vi "Solar_V4.vi"() -> ()   [LabVIEW 2012]
uses:
  <vilib>/Utility/file.llb/Write To Spreadsheet File (string).vi
panel:
  out "DSSC1_WP 3":dbl
  out "DSSC1_WP 2":dbl
  out "DSSC3_WP":dbl
  out "POLYSI1_WP":dbl
  out "THINFILM1_WP":dbl
  out "DSSC1_WP":dbl
  out "THINFILM2_WP":dbl
  out "POLYSI2_WP":dbl
  out "DSSC2_WP":dbl
  out "Wind Angle":sgl(knob) scale=0.0..360.0
  out "Wind Speed Speed":i16(knob) scale=0.0..100.0
  out "?":string
  out "inside":dbl(slide) scale=-10.0..50.0
  out "outside":dbl(slide) scale=-10.0..50.0
  in  "EXIT":bool
  out "LED":bool
  in  "stop":bool
  out "Energy":dbl format="%#.3f"
  out "Power":dbl format="%#.3f"
  out "Current":dbl format="%#.3f"
  out "Voltage":dbl format="%#.3f"
  out "Energy":dbl format="%#.3f"
  out "Power":dbl format="%#.3f"
  out "Current":dbl format="%#.3f"
  out "Voltage":dbl format="%#.3f"
  out "Energy":dbl format="%#.3f"
  out "Power":dbl format="%#.3f"
  out "Current":dbl format="%#.3f"
  out "Voltage":dbl format="%#.3f"
  out "Energy":dbl format="%#.3f"
  out "Power":dbl format="%#.3f"
  out "Current":dbl format="%#.3f"
  out "Voltage":dbl format="%#.3f"
  out "Energy":dbl format="%#.3f"
  out "Power":dbl format="%#.3f"
  out "Current":dbl format="%#.3f"
  out "Voltage":dbl format="%#.3f"
  out "Energy":dbl format="%#.3f"
  out "Power":dbl format="%#.3f"
  out "Current":dbl format="%#.3f"
  out "Voltage":dbl format="%#.3f"
  out "Energy":dbl format="%#.3f"
  out "Power":dbl format="%#.3f"
  out "Current":dbl format="%#.3f"
  out "Voltage":dbl format="%#.3f"
  out "Poly Si 1":dbl=1.3668
  out "Poly Si 2":dbl=1.3668
  out "Thin film 2":dbl=1.3668
  out "thin Film 1":dbl=1.3668
  out "DSSC3":dbl=1.0
  out "DSSC 2":dbl=0.01296
  out "DSSC 1":dbl=0.375
  out "Waveform Chart":dynamicdata(graph)
  in  "Solar Related":T1(tab)
  out "Solar Tilted":dynamicdata(graph)
  out "Solar vertical":dynamicdata(graph)
  out "Solar Tracked":dynamicdata(graph)
  out "Solar Meteo":dynamicdata(graph)
  out "Solar UV":dynamicdata(graph)
  in  "TEMPERATURES":T2(tab)
  out "Temperature DSSC 1":dynamicdata(graph)
  out "Temperature DSSC 2":dynamicdata(graph)
  out "Temperature Poly Si":dynamicdata(graph)
  out "Temperature Thin Film":dynamicdata(graph)
  out "Array":dbl[][](array[numeric])
  # "DSSC 1"
  # "DSSC 2"
  # "DSSC 3"
  # "Poly Si 1"
  # "Poly Si 2"
  # "Thin Film 1"
  # "Thin Film 2"
  # "Temperatures"
  # "Weather Station"
  # "DSSC 1"
  # "DSSC 2"
  # "DSSC 3"
  # "Poly Si 1"
  # "Poly Si  2"
  # "Thin Film 1"
  # "Thin Film 2"
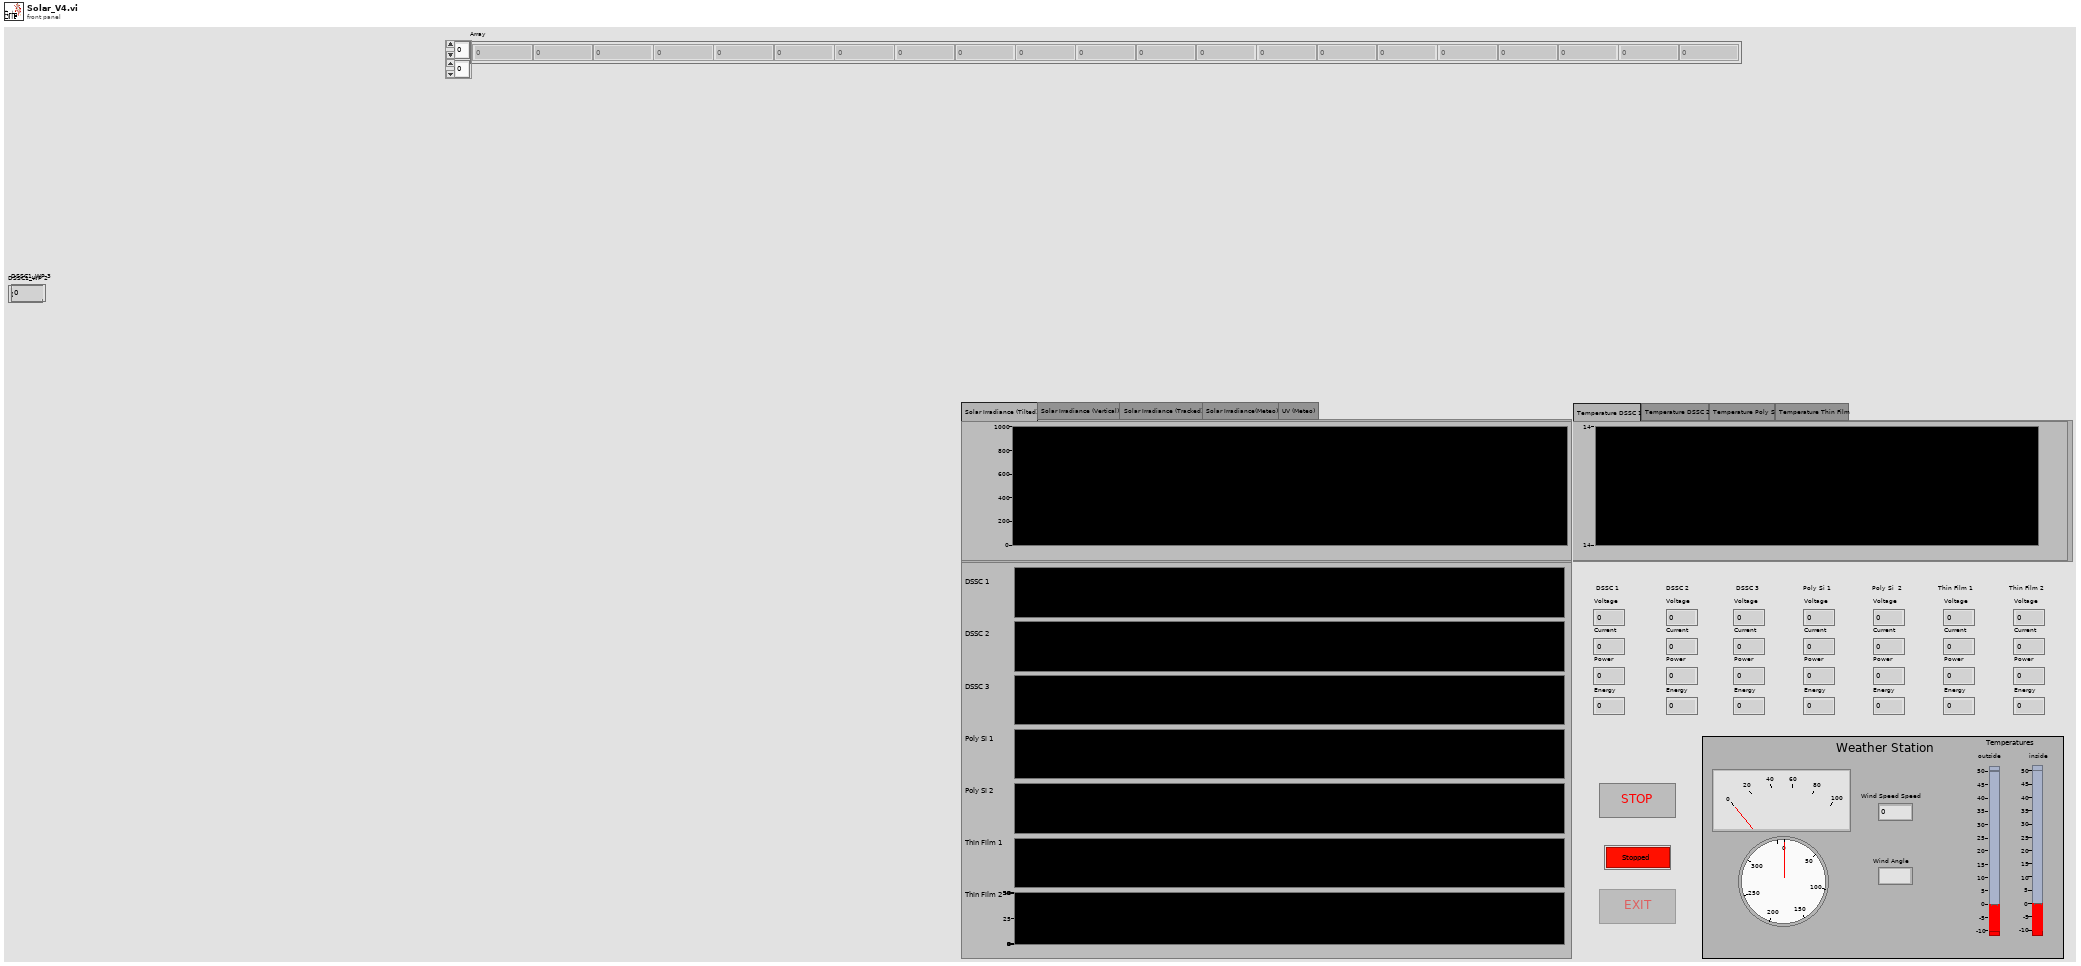
[diagram p1: front panel]
types:
  T1 = enum32{"Solar Irradiance (Tilted)", "Solar Irradiance (Vertical)", "Solar Irradiance (Tracked)", "Solar Irradiance(Meteo)", "UV (Meteo)"}
  T2 = enum32{"Temperature DSSC 1", "Temperature DSSC 2", "Temperature Poly Si", "Temperature Thin Film"}
  T3 = enum8{"Enabled", "Disabled", "Disabled and Grayed Out"}
  T4 = enum16{"open", "replace", "create", "open or create", "replace or create", "replace or create with confirmation"}
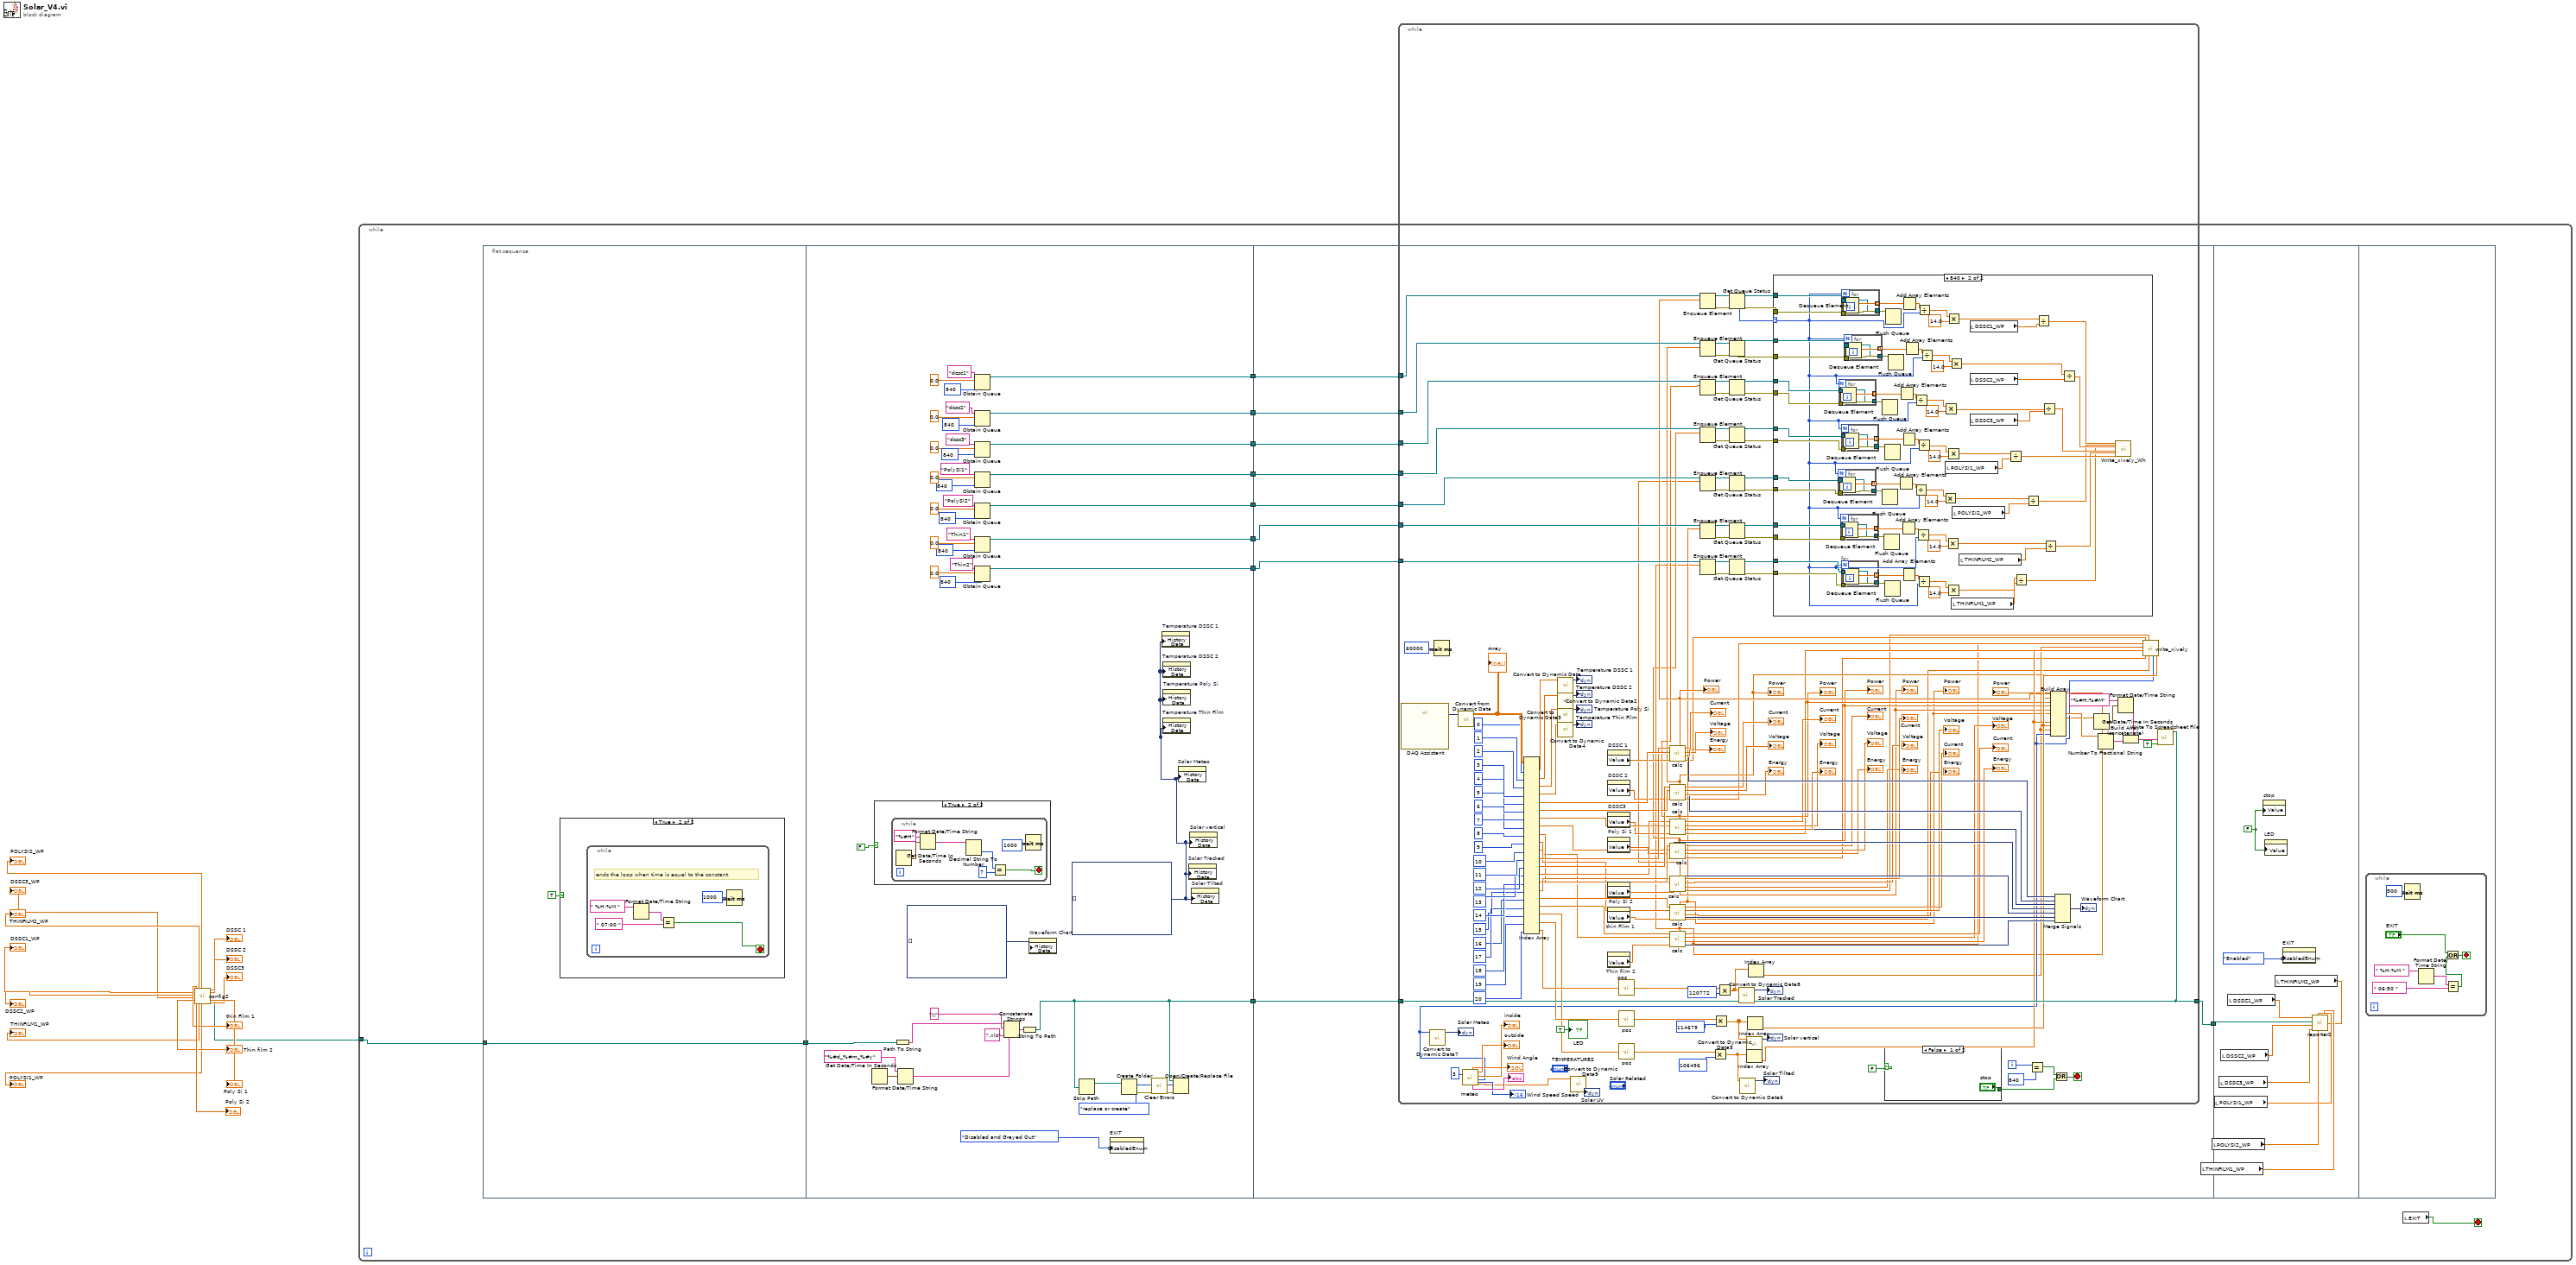
[diagram p0: block diagram]
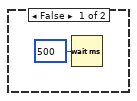
[diagram p3: hidden frame]
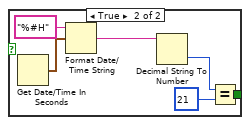
[diagram p5: hidden frame]
diagram:
  n1 = call "config2.vi"() -> ("thin Film 1"=→"thin Film 1":dbl, "DSSC1_WP"=→"DSSC1_WP":dbl, "DSSC2_WP"=→"DSSC2_WP":dbl, "DSSC3_WP"=→"DSSC3_WP":dbl, "thin Film 2"=→"Thin film 2":dbl, "Poly Si 2"=→"Poly Si 2":dbl, "THINFILM2_WP"=→"THINFILM2_WP":dbl, "THINFILM1_WP"=→"THINFILM1_WP":dbl, "POLYSI2_WP"=→"POLYSI2_WP":dbl, "POLYSI1_WP"=→"POLYSI1_WP":dbl, "Poly Si 1"=→"Poly Si 1":dbl, "DSSC 2"=→"DSSC 2":dbl, "DSSC 1"=→"DSSC 1":dbl, "path"=w8:path, "DSSC3"=→"DSSC3":dbl)  [unwired: 5 in]
  n2 = while {
    tunnel: w8 -> [w17]
    stop <- w16 stop-if-true
    n3 = flat-sequence {
      tunnel: [w29] -> w27
      tunnel: w17 -> [w29]
      tunnel: w27 -> [w38]
      tunnel: [w37] -> w26
      tunnel: [w52] -> w25
      tunnel: [w51] -> w24
      tunnel: [w50] -> w23
      tunnel: [w49] -> w22
      tunnel: [w48] -> w21
      tunnel: [w47] -> w20
      tunnel: [w46] -> w19
      tunnel: w26 -> [w96]
      tunnel: [w95] -> w18
      tunnel: w25 -> [w89]
      tunnel: w24 -> [w88]
      tunnel: w23 -> [w94]
      tunnel: w22 -> [w93]
      tunnel: w21 -> [w92]
      tunnel: w20 -> [w91]
      tunnel: w19 -> [w90]
      tunnel: w18 -> [w400]
      frame #0 {
        n4 = case shown="True" TRUE {
          frame False {
          }
          frame True {
            n5 = while {
              stop <- w30 stop-if-true
              # "ends the loop when time is equal to the constant"
              n6 = Format Date/Time String(time format string (%c)=" %H:%M ") -> (date/time string=w31:string)  [unwired: 2 in]
              n7 = Equal?(x=w31, y=" 07:00 " ("time format string (%c)")) -> (x = y?=w30:bool)
              n8 = Wait (ms)(milliseconds to wait=u32 1000) -> ()  [unwired: 1 out]
            }
          }
        }
      }
      frame #1 {
        w35 = dynamicdata[] [] ("History Data")
        n9 = Get Date/Time In Seconds() -> (seconds since 1Jan1904=w39:timestamp)
        n10 = case shown="True" FALSE {
          frame False {
            n11 = Wait (ms)(milliseconds to wait=u32 500) -> ()  [unwired: 1 out]
          }
          frame True {
            n12 = while {
              stop <- w81 stop-if-true
              n13 = Get Date/Time In Seconds() -> (seconds since 1Jan1904=w87:timestamp)
              n14 = Format Date/Time String(time format string (%c)="%#H", seconds (now)=w87) -> (date/time string=w84:string)  [unwired: 1 in]
              n15 = Decimal String To Number(string=w84) -> (number=w83:i32)  [unwired: 2 in, 1 out]
              n16 = Equal?(x=w83, y=7) -> (x = y?=w81:bool)
              n17 = Wait (ms)(milliseconds to wait=u32 1000) -> ()  [unwired: 1 out]
            }
          }
        }
        n18 = Path To String(path=w38) -> (string=w43:string)
        n19 = Format Date/Time String(time format string (%c)="%#d_%#m_%#y", seconds (now)=w39) -> (date/time string=w41:string)  [unwired: 1 in]
        n20 = Obtain Queue(max queue size (-1, unlimited)=840, name (unnamed)="dcsc1", element data type=0.0) -> (queue out=w52:refnum<queue>)  [unwired: 2 in, 2 out]
        n21 = Obtain Queue(max queue size (-1, unlimited)=840, name (unnamed)="dcsc2", element data type=0.0) -> (queue out=w51:refnum<queue>)  [unwired: 2 in, 2 out]
        n22 = Obtain Queue(max queue size (-1, unlimited)=840, name (unnamed)="dcsc3", element data type=0.0) -> (queue out=w50:refnum<queue>)  [unwired: 2 in, 2 out]
        n23 = Obtain Queue(max queue size (-1, unlimited)=840, name (unnamed)="PolySI1", element data type=0.0) -> (queue out=w49:refnum<queue>)  [unwired: 2 in, 2 out]
        n24 = Obtain Queue(max queue size (-1, unlimited)=840, name (unnamed)="PolySI2", element data type=0.0) -> (queue out=w48:refnum<queue>)  [unwired: 2 in, 2 out]
        n25 = Obtain Queue(max queue size (-1, unlimited)=840, name (unnamed)="Thin1", element data type=0.0) -> (queue out=w47:refnum<queue>)  [unwired: 2 in, 2 out]
        n26 = Obtain Queue(max queue size (-1, unlimited)=840, name (unnamed)="Thin2", element data type=0.0) -> (queue out=w46:refnum<queue>)  [unwired: 2 in, 2 out]
        n27 = Concatenate Strings(w43, "\\" ("string"), w41, ".xls" ("string")) -> (w45:string)
        n28 = String To Path(string=w45) -> (path=w37:path)
        n29 = property on="Waveform Chart" class="WFChart (strict)"("History Data"=dynamicdata[] []) -> ()  [unwired: 2 in, 2 out]
        n30 = Strip Path(path=w37) -> (stripped path=w78:path)  [unwired: 1 out]
        n31 = property on="EXIT" class="Bool (strict)"("DisabledEnum"=T3."Disabled and Grayed Out" ("Disabled")) -> ()  [unwired: 2 in, 2 out]
        n32 = Create Folder(path (use dialog)=w78) -> (error out=w77:errorcluster)  [unwired: 2 in, 2 out]
        n33 = call <vilib>:"Clear Errors.vi"("error in (no error)"=w77) -> ("error out"=w76:errorcluster)  [unwired: 6 in]
        n34 = property on="Temperature DSSC 1" class="WFChart (strict)"("History Data"=w35) -> ()  [unwired: 2 in, 2 out]
        n35 = property on="Temperature DSSC 2" class="WFChart (strict)"("History Data"=w35) -> ()  [unwired: 2 in, 2 out]
        n36 = property on="Temperature Thin Film" class="WFChart (strict)"("History Data"=w35) -> ()  [unwired: 2 in, 2 out]
        n37 = property on="Temperature Poly Si" class="WFChart (strict)"("History Data"=w35) -> ()  [unwired: 2 in, 2 out]
        n38 = Open/Create/Replace File(file path (use dialog)=w37, error in=w76, operation (0:open)=T4."replace or create") -> ()  [unwired: 3 in, 3 out]
        n39 = property on="Solar Meteo" class="WFChart (strict)"("History Data"=w35) -> ()  [unwired: 2 in, 2 out]
        n40 = property on="Solar Tracked" class="WFChart (strict)"("History Data"=w35) -> ()  [unwired: 2 in, 2 out]
        n41 = property on="Solar vertical" class="WFChart (strict)"("History Data"=w35) -> ()  [unwired: 2 in, 2 out]
        n42 = property on="Solar Tilted" class="WFChart (strict)"("History Data"=w35) -> ()  [unwired: 2 in, 2 out]
      }
      frame #2 {
        n43 = while {
          tunnel: w96 -> [w245]
          tunnel: [w245] -> w95
          tunnel: w94 -> [w116]
          tunnel: w93 -> [w115]
          tunnel: w92 -> [w114]
          tunnel: w91 -> [w113]
          tunnel: w90 -> [w112]
          tunnel: w89 -> [w118]
          tunnel: w88 -> [w117]
          i -> [w152]
          stop <- w148 stop-if-true
          n44 = call "DAQ Assistant"() -> ("data"=w246:dynamicdata)  [unwired: 17 in, 2 out]
          n45 = Wait (ms)(milliseconds to wait=u32 60000) -> ()  [unwired: 1 out]
          n46 = call "Convert from Dynamic Data"("Dynamic Data Type"=w246) -> ("Array"=w270:dbl[][])  [unwired: 3 in]
          "Array" <- w270
          n47 = call "meteo.vi"("ComPort 2"=i16 3) -> ("Wind Speed 2"=→"Wind Speed Speed":i16, "Wind Angle 2"=→"Wind Angle":sgl, "Direction 2"=→"?":string, "Outside Temperature"=→"outside":sgl, "Inside Temp"=→"inside":sgl, "Solar"=w156:i16, "UV"=w153:sgl)
          n48 = call "Convert to Dynamic Data7"("Double"=w156) -> ("Dynamic Data Type"=→"Solar Meteo":dynamicdata)  [unwired: 3 in]
          n49 = Index Array(array=w270, index (col) #1=0 ("index (row)"), index (col) #2=1 ("index (col)"), index (col) #3=2 ("index (col)"), index (col) #4=3 ("index (col)"), index (col) #5=4 ("index (col)"), index (col) #6=5 ("index (col)"), index (col) #7=6 ("index (col)"), index (col) #8=7 ("index (col)"), index (col) #9=8 ("index (col)"), index (col) #10=9 ("index (col)"), index (col) #11=10 ("index (col)"), index (col) #12=11 ("index (col)"), index (col) #13=12 ("index (col)"), index (col) #14=13 ("index (col)"), index (col) #15=14 ("index (col)"), index (col) #16=15 ("index (col)"), index (col) #17=16 ("index (col)"), index (col) #18=17 ("index (col)"), index (col) #19=18 ("index (col)"), index (col) #20=19 ("index (col)"), index (col) #21=20 ("index (col)")) -> (element #1=w187:dbl[], element #2=w186:dbl[], element #3=w185:dbl[], element #4=w184:dbl[], element #5=w237:dbl[], element #6=w227:dbl[], element #7=w224:dbl[], element #8=w220:dbl[], element #9=w202:dbl[], element #10=w201:dbl[], element #11=w200:dbl[], element #12=w236:dbl[], element #13=w226:dbl[], element #14=w225:dbl[], element #15=w206:dbl[], element #16=w205:dbl[], element #17=w204:dbl[], element #18=w203:dbl[], element #19=w171:dbl[], element #20=w172:dbl[], element #21=w207:dbl[])  [unwired: 21 in]
          n50 = call "Convert to Dynamic Data"("Array"=w187) -> ("Dynamic Data Type"=→"Temperature DSSC 1":dynamicdata)  [unwired: 3 in]
          n51 = call "Convert to Dynamic Data2"("Array"=w186) -> ("Dynamic Data Type"=→"Temperature DSSC 2":dynamicdata)  [unwired: 3 in]
          n52 = call "Convert to Dynamic Data3"("Array"=w185) -> ("Dynamic Data Type"=→"Temperature Poly Si":dynamicdata)  [unwired: 3 in]
          n53 = call "Convert to Dynamic Data4"("Array"=w184) -> ("Dynamic Data Type"=→"Temperature Thin Film":dynamicdata)  [unwired: 3 in]
          n54 = call "Convert to Dynamic Data9"("Double"=w153) -> ("Dynamic Data Type"=→"Solar UV":dynamicdata)  [unwired: 3 in]
          n55 = property on="DSSC 1" class="DigNum (strict)"() -> ("Value"=w183:dbl)  [unwired: 2 in, 2 out]
          n56 = property on="DSSC 2" class="DigNum (strict)"() -> ("Value"=w182:dbl)  [unwired: 2 in, 2 out]
          n57 = property on="DSSC3" class="DigNum (strict)"() -> ("Value"=w181:dbl)  [unwired: 2 in, 2 out]
          n58 = property on="Poly Si 1" class="DigNum (strict)"() -> ("Value"=w178:dbl)  [unwired: 2 in, 2 out]
          n59 = property on="Poly Si 2" class="DigNum (strict)"() -> ("Value"=w177:dbl)  [unwired: 2 in, 2 out]
          n60 = property on="thin Film 1" class="DigNum (strict)"() -> ("Value"=w180:dbl)  [unwired: 2 in, 2 out]
          n61 = property on="Thin film 2" class="DigNum (strict)"() -> ("Value"=w179:dbl)  [unwired: 2 in, 2 out]
          n62 = call "pos.vi"("Input"=w207) -> ("Output"=w244:dbl[])
          n63 = call "pos.vi"("Input"=w172) -> ("Output"=w175:dbl[])
          n64 = call "pos.vi"("Input"=w171) -> ("Output"=w173:dbl[])
          n65 = call "calc.vi"("Input Current"=w236, "Input voltage"=w237, "Area factor"=w183) -> ("Waveform Chart"=w233:dynamicdata, "Power"=w109:dbl, "Current"=→"Current":dbl, "Voltage"=→"Voltage":dbl, "Energy"=→"Energy":dbl, "Power(m2)"=w108:dbl)
          "Power" <- w109
          n66 = call "calc.vi"("Input Current"=w226, "Input voltage"=w227, "Area factor"=w182) -> ("Waveform Chart"=w228:dynamicdata, "Power"=w107:dbl, "Current"=→"Current":dbl, "Voltage"=→"Voltage":dbl, "Energy"=→"Energy":dbl, "Power(m2)"=w106:dbl)
          "Power" <- w107
          n67 = call "calc.vi"("Input Current"=w225, "Input voltage"=w224, "Area factor"=w181) -> ("Waveform Chart"=w221:dynamicdata, "Power"=w105:dbl, "Current"=→"Current":dbl, "Voltage"=→"Voltage":dbl, "Energy"=→"Energy":dbl, "Power(m2)"=w104:dbl)
          "Power" <- w105
          n68 = call "calc.vi"("Input Current"=w206, "Input voltage"=w220, "Area factor"=w178) -> ("Waveform Chart"=w219:dynamicdata, "Power"=w103:dbl, "Current"=→"Current":dbl, "Voltage"=→"Voltage":dbl, "Energy"=→"Energy":dbl, "Power(m2)"=w100:dbl)
          "Power" <- w103
          n69 = call "calc.vi"("Input Current"=w205, "Input voltage"=w202, "Area factor"=w177) -> ("Waveform Chart"=w199:dynamicdata, "Power"=w102:dbl, "Current"=→"Current":dbl, "Voltage"=→"Voltage":dbl, "Energy"=→"Energy":dbl, "Power(m2)"=w101:dbl)
          "Power" <- w102
          n70 = call "calc.vi"("Input Current"=w204, "Input voltage"=w201, "Area factor"=w180) -> ("Waveform Chart"=w198:dynamicdata, "Power"=w99:dbl, "Current"=→"Current":dbl, "Voltage"=→"Voltage":dbl, "Energy"=→"Energy":dbl, "Power(m2)"=w98:dbl)
          "Power" <- w99
          n71 = call "calc.vi"("Input Current"=w203, "Input voltage"=w200, "Area factor"=w179) -> ("Waveform Chart"=w197:dynamicdata, "Power"=w97:dbl, "Current"=→"Current":dbl, "Voltage"=→"Voltage":dbl, "Energy"=→"Energy":dbl)  [unwired: 1 out]
          "Power" <- w97
          n72 = Enqueue Element(queue=w118, element=w109) -> (queue out=w120:refnum<queue>, error out=w122:errorcluster)  [unwired: 2 in, 1 out]
          n73 = Enqueue Element(queue=w117, element=w107) -> (queue out=w124:refnum<queue>, error out=w125:errorcluster)  [unwired: 2 in, 1 out]
          n74 = Enqueue Element(queue=w116, element=w105) -> (queue out=w128:refnum<queue>, error out=w129:errorcluster)  [unwired: 2 in, 1 out]
          n75 = Enqueue Element(queue=w115, element=w103) -> (queue out=w130:refnum<queue>, error out=w131:errorcluster)  [unwired: 2 in, 1 out]
          n76 = Enqueue Element(queue=w114, element=w102) -> (queue out=w132:refnum<queue>, error out=w133:errorcluster)  [unwired: 2 in, 1 out]
          n77 = Enqueue Element(queue=w113, element=w99) -> (queue out=w134:refnum<queue>, error out=w135:errorcluster)  [unwired: 2 in, 1 out]
          n78 = Enqueue Element(queue=w112, element=w97) -> (queue out=w136:refnum<queue>, error out=w137:errorcluster)  [unwired: 2 in, 1 out]
          n79 = Multiply(x=w173, y=106496) -> (x*y=w166:dbl[])
          n80 = Multiply(x=w175, y=114679) -> (x*y=w167:dbl[])
          n81 = Multiply(x=w244, y=120772) -> (x*y=w168:dbl[])
          n82 = Get Queue Status(queue=w120, error in (no error)=w122) -> (queue out=w121:refnum<queue>, error out=w123:errorcluster, # elements in queue=w119:i32)  [unwired: 1 in, 5 out]
          n83 = Get Queue Status(queue=w124, error in (no error)=w125) -> (queue out=w126:refnum<queue>, error out=w127:errorcluster)  [unwired: 1 in, 6 out]
          n84 = Get Queue Status(queue=w128, error in (no error)=w129) -> (queue out=w138:refnum<queue>, error out=w139:errorcluster)  [unwired: 1 in, 6 out]
          n85 = Get Queue Status(queue=w130, error in (no error)=w131) -> (queue out=w140:refnum<queue>, error out=w141:errorcluster)  [unwired: 1 in, 6 out]
          n86 = Get Queue Status(queue=w132, error in (no error)=w133) -> (queue out=w142:refnum<queue>, error out=w143:errorcluster)  [unwired: 1 in, 6 out]
          n87 = Get Queue Status(queue=w134, error in (no error)=w135) -> (queue out=w144:refnum<queue>, error out=w145:errorcluster)  [unwired: 1 in, 6 out]
          n88 = Get Queue Status(queue=w136, error in (no error)=w137) -> (queue out=w146:refnum<queue>, error out=w147:errorcluster)  [unwired: 1 in, 6 out]
          n89 = call "Convert to Dynamic Data8"("Array"=w168) -> ("Dynamic Data Type"=→"Solar Tracked":dynamicdata)  [unwired: 3 in]
          n90 = call "Convert to Dynamic Data6"("Array"=w166) -> ("Dynamic Data Type"=→"Solar Tilted":dynamicdata)  [unwired: 3 in]
          n91 = call "Convert to Dynamic Data5"("Array"=w167) -> ("Dynamic Data Type"=→"Solar vertical":dynamicdata)  [unwired: 3 in]
          n92 = Index Array(array=w166) -> (element=w157:dbl)  [unwired: 1 in]
          n93 = Index Array(array=w167) -> (element=w158:dbl)  [unwired: 1 in]
          n94 = Index Array(array=w168) -> (element=w110:dbl)  [unwired: 1 in]
          n95 = case shown="840" w119 {
            selector: w119 -> [_ w292]
            tunnel: w121 -> [_ w348]
            tunnel: w123 -> [_ w344]
            tunnel: w126 -> [_ w334]
            tunnel: w127 -> [_ w333]
            tunnel: w138 -> [_ w302]
            tunnel: w139 -> [_ w301]
            tunnel: w140 -> [_ w300]
            tunnel: w141 -> [_ w299]
            tunnel: w142 -> [_ w298]
            tunnel: w143 -> [_ w297]
            tunnel: w144 -> [_ w296]
            tunnel: w145 -> [_ w295]
            tunnel: w146 -> [_ w294]
            tunnel: w147 -> [_ w293]
            frame 0, Default {
            }
            frame 840 {
              n96 = for {
                N: w292 -> [_]
                tunnel: w298 -> [w363]
                tunnel: [w362] -> w320 mode=indexing
                tunnel: [w361] -> w319
                tunnel: [w360] -> w318
                tunnel: w297 -> [w359]
                n97 = Dequeue Element(queue=w363, error in (no error)=w359) -> (queue out=w360:refnum<queue>, element=w362:dbl, error out=w361:errorcluster)  [unwired: 1 in, 1 out]
              }
              n98 = for {
                N: w292 -> [_]
                tunnel: w302 -> [w373]
                tunnel: [w372] -> w332 mode=indexing
                tunnel: [w371] -> w331
                tunnel: [w370] -> w330
                tunnel: w301 -> [w369]
                n99 = Dequeue Element(queue=w373, error in (no error)=w369) -> (queue out=w370:refnum<queue>, element=w372:dbl, error out=w371:errorcluster)  [unwired: 1 in, 1 out]
              }
              n100 = for {
                N: w292 -> [_]
                tunnel: w296 -> [w358]
                tunnel: [w357] -> w314 mode=indexing
                tunnel: [w356] -> w313
                tunnel: [w355] -> w312
                tunnel: w295 -> [w354]
                n101 = Dequeue Element(queue=w358, error in (no error)=w354) -> (queue out=w355:refnum<queue>, element=w357:dbl, error out=w356:errorcluster)  [unwired: 1 in, 1 out]
              }
              n102 = for {
                N: w292 -> [_]
                tunnel: w300 -> [w368]
                tunnel: [w367] -> w326 mode=indexing
                tunnel: [w366] -> w325
                tunnel: [w365] -> w324
                tunnel: w299 -> [w364]
                n103 = Dequeue Element(queue=w368, error in (no error)=w364) -> (queue out=w365:refnum<queue>, element=w367:dbl, error out=w366:errorcluster)  [unwired: 1 in, 1 out]
              }
              n104 = for {
                N: w292 -> [_]
                tunnel: w294 -> [w353]
                tunnel: [w352] -> w308 mode=indexing
                tunnel: [w351] -> w307
                tunnel: [w350] -> w306
                tunnel: w293 -> [w349]
                n105 = Dequeue Element(queue=w353, error in (no error)=w349) -> (queue out=w350:refnum<queue>, element=w352:dbl, error out=w351:errorcluster)  [unwired: 1 in, 1 out]
              }
              n106 = for {
                N: w292 -> [_]
                tunnel: w348 -> [w383]
                tunnel: [w382] -> w347 mode=indexing
                tunnel: [w381] -> w346
                tunnel: [w380] -> w345
                tunnel: w344 -> [w379]
                n107 = Dequeue Element(queue=w383, error in (no error)=w379) -> (queue out=w380:refnum<queue>, element=w382:dbl, error out=w381:errorcluster)  [unwired: 1 in, 1 out]
              }
              n108 = for {
                N: w292 -> [_]
                tunnel: w334 -> [w378]
                tunnel: [w377] -> w340 mode=indexing
                tunnel: [w376] -> w339
                tunnel: [w375] -> w338
                tunnel: w333 -> [w374]
                n109 = Dequeue Element(queue=w378, error in (no error)=w374) -> (queue out=w375:refnum<queue>, element=w377:dbl, error out=w376:errorcluster)  [unwired: 1 in, 1 out]
              }
              n110 = Flush Queue(queue=w318, error in (no error)=w319) -> ()  [unwired: 3 out]
              n111 = Flush Queue(queue=w330, error in (no error)=w331) -> ()  [unwired: 3 out]
              n112 = Flush Queue(queue=w312, error in (no error)=w313) -> ()  [unwired: 3 out]
              n113 = Flush Queue(queue=w324, error in (no error)=w325) -> ()  [unwired: 3 out]
              n114 = Flush Queue(queue=w306, error in (no error)=w307) -> ()  [unwired: 3 out]
              n115 = Flush Queue(queue=w345, error in (no error)=w346) -> ()  [unwired: 3 out]
              n116 = Flush Queue(queue=w338, error in (no error)=w339) -> ()  [unwired: 3 out]
              n117 = Add Array Elements(numeric array=w320) -> (sum=w317:dbl)
              n118 = Add Array Elements(numeric array=w332) -> (sum=w329:dbl)
              n119 = Add Array Elements(numeric array=w314) -> (sum=w311:dbl)
              n120 = Add Array Elements(numeric array=w326) -> (sum=w323:dbl)
              n121 = Add Array Elements(numeric array=w308) -> (sum=w305:dbl)
              n122 = Add Array Elements(numeric array=w347) -> (sum=w343:dbl)
              n123 = Add Array Elements(numeric array=w340) -> (sum=w337:dbl)
              n124 = Divide(x=w317, y=w292) -> (x/y=w316:dbl)
              n125 = Divide(x=w329, y=w292) -> (x/y=w328:dbl)
              n126 = Divide(x=w311, y=w292) -> (x/y=w310:dbl)
              n127 = Divide(x=w323, y=w292) -> (x/y=w322:dbl)
              n128 = Divide(x=w305, y=w292) -> (x/y=w304:dbl)
              n129 = Divide(x=w343, y=w292) -> (x/y=w342:dbl)
              n130 = Divide(x=w337, y=w292) -> (x/y=w336:dbl)
              n131 = Multiply(x=w316, y=14.0) -> (x*y=w279:dbl)
              n132 = Multiply(x=w328, y=14.0) -> (x*y=w285:dbl)
              n133 = local read "POLYSI1_WP"() -> (w280:dbl)
              n134 = Multiply(x=w310, y=14.0) -> (x*y=w276:dbl)
              n135 = Multiply(x=w322, y=14.0) -> (x*y=w282:dbl)
              n136 = Multiply(x=w304, y=14.0) -> (x*y=w272:dbl)
              n137 = Multiply(x=w342, y=14.0) -> (x*y=w291:dbl)
              n138 = Multiply(x=w336, y=14.0) -> (x*y=w288:dbl)
              n139 = local read "THINFILM1_WP"() -> (w273:dbl)
              n140 = local read "POLYSI2_WP"() -> (w277:dbl)
              n141 = local read "THINFILM2_WP"() -> (w274:dbl)
              n142 = local read "DSSC1_WP"() -> (w289:dbl)
              n143 = local read "DSSC2_WP"() -> (w286:dbl)
              n144 = local read "DSSC3_WP"() -> (w284:dbl)
              n145 = Divide(x=w282, y=w280) -> (x/y=w281:dbl)
              n146 = Divide(x=w272, y=w273) -> (x/y=w271:dbl)
              n147 = Divide(x=w279, y=w277) -> (x/y=w278:dbl)
              n148 = Divide(x=w291, y=w289) -> (x/y=w290:dbl)
              n149 = Divide(x=w285, y=w284) -> (x/y=w283:dbl)
              n150 = Divide(x=w276, y=w274) -> (x/y=w275:dbl)
              n151 = Divide(x=w288, y=w286) -> (x/y=w287:dbl)
              n152 = call "Write_xively_Wh.vi"("thinfilm2"=w271, "Thinfilm1"=w275, "Poly Si 2"=w278, "Poly Si 1"=w281, "DSSC3"=w283, "DSSC2"=w287, "DSSC1"=w290) -> ()  [unwired: 5 in]
            }
          }
          n153 = case shown="False" FALSE {
            tunnel: ["stop" w385] -> w149
            frame False {
            }
            frame True {
              n154 = Get Date/Time In Seconds() -> (seconds since 1Jan1904=w390:timestamp)
              n155 = Format Date/Time String(time format string (%c)="%#H", seconds (now)=w390) -> (date/time string=w388:string)  [unwired: 1 in]
              n156 = Decimal String To Number(string=w388) -> (number=w387:i32)  [unwired: 2 in, 1 out]
              n157 = Equal?(x=w387, y=21) -> (x = y?=w385:bool)
            }
          }
          n158 = Equal?(x=w152, y=840) -> (x = y?=w150:bool)
          n159 = Build Array(w109, w107, w105, w103, w102, w99, w97, w157, w158, w110, w156) -> (w249:dbl[])
          n160 = Or(x=w150, y=w149) -> (x .or. y?=w148:bool)
          n161 = Merge Signals(w233, w228, w221, w219, w199, w198, w197) -> (→"Waveform Chart":dynamicdata)
          n162 = Get Date/Time In Seconds() -> (seconds since 1Jan1904=w253:timestamp)
          n163 = Number To Fractional String(number=w249) -> (F-format string=w250:string[])  [unwired: 3 in]
          n164 = Format Date/Time String(time format string (%c)="%#H:%#M", seconds (now)=w253) -> (date/time string=w251:string)  [unwired: 1 in]
          n165 = Build Array (concatenate)(w251, w250) -> (w248:string[])
          n166 = call "write_xively.vi"("Solar__Tilted_"=w157, "Solar__Tracked_"=w110, "Solar__Vertical_"=w158, "Solar__meteo_"=w156, "Thin_Film_2"=w97, "Thin_Film_1"=w98, "Poly Si 2"=w101, "Poly Si 1"=w100, "DSSC3"=w104, "DSSC2"=w106, "DSSC1"=w108) -> ()  [unwired: 1 in]
          n167 = call-poly <vilib>:"Write To Spreadsheet File.vi"("append to file? (new file:F)"=TRUE, "1D data"=w248, "file path (dialog if empty)"=w245) -> ()  [unwired: 5 in, 1 out]
          "LED" <- TRUE
        }
      }
      frame #3 {
        w398 = FALSE ("stop")
        n168 = local read "THINFILM1_WP"() -> (w392:dbl)
        n169 = local read "POLYSI2_WP"() -> (w394:dbl)
        n170 = local read "POLYSI1_WP"() -> (w395:dbl)
        n171 = local read "DSSC3_WP"() -> (w393:dbl)
        n172 = local read "DSSC2_WP"() -> (w396:dbl)
        n173 = local read "DSSC1_WP"() -> (w397:dbl)
        n174 = property on="stop" class="Bool (strict)"("Value"=w398) -> ()  [unwired: 2 in, 2 out]
        n175 = property on="LED" class="Bool (strict)"("Value"=w398) -> ()  [unwired: 2 in, 2 out]
        n176 = local read "THINFILM2_WP"() -> (w391:dbl)
        n177 = property on="EXIT" class="Bool (strict)"("DisabledEnum"=T3."Enabled" ("Disabled")) -> ()  [unwired: 2 in, 2 out]
        n178 = call "reporter2.vi"("DSSC1_Wp"=w397, "PolySI1_wp"=w395, "file path (dialog if empty)"=w400, "DSSC2_WP"=w396, "Polysi2_wp"=w394, "DSSC3_Wp"=w393, "Thin1Wp"=w392, "Thin2Wp"=w391) -> ()  [unwired: 1 out]
      }
      frame #4 {
        n179 = while {
          stop <- w401 stop-if-true
          n180 = Wait (ms)(milliseconds to wait=u32 500) -> ()  [unwired: 1 out]
          n181 = Format Date/Time String(time format string (%c)=" %H:%M ") -> (date/time string=w404:string)  [unwired: 2 in]
          n182 = Equal?(x=w404, y=" 06:50 " ("time format string (%c)")) -> (x = y?=w402:bool)
          n183 = Or(x="EXIT", y=w402) -> (x .or. y?=w401:bool)
        }
      }
    }
    n184 = local read "EXIT"() -> (w16:bool)
  }
